vi "DAQ_AI_Chans.vi"(3 "error in":errorcluster, 5 "DAQ Settings":T1={"Shutters Settings"=[{"Name"="Shutter 1", "DAQ Channel/line"="Dev1/port0/line0", "Active"=FALSE}, {"Name"="Shutter 2", "DAQ Channel/line"="Dev1/port0/line1", "Active"=FALSE}], "Shutter Task"="", "Acquire Settings"=[], "AI Task"="", "Sample mode"=10178, "Number of Samples"=0, "Rate"=0.0, "AI Name"="", "DO Name"=""} {"Sample mode" items=["Finite Samples"=10178, "Continuous Samples"=10123, "Hardware Timed Single Point"=12522]; "Acquire Settings"."input terminal configuration" items=["default"=-1, "RSE"=10083, "NRSE"=10078, "Differential"=10106, "Pseudodifferential"=12529]}) -> (0 "error out":errorcluster, 2 "Acquire Out":refnum<k21>)   [LabVIEW 2020]
uses:
  Type defs/DAQ_set_Ctrl.ctl
  Type defs/DAQ_Shutter_Ctrl.ctl
  Type defs/DAQ_AI_Ctrl.ctl
  <vilib>/DAQmx/create/channels.llb/DAQmx Create Channel (AI-Voltage-Basic).vi
  <vilib>/DAQmx/configure/timing.llb/DAQmx Timing (Sample Clock).vi
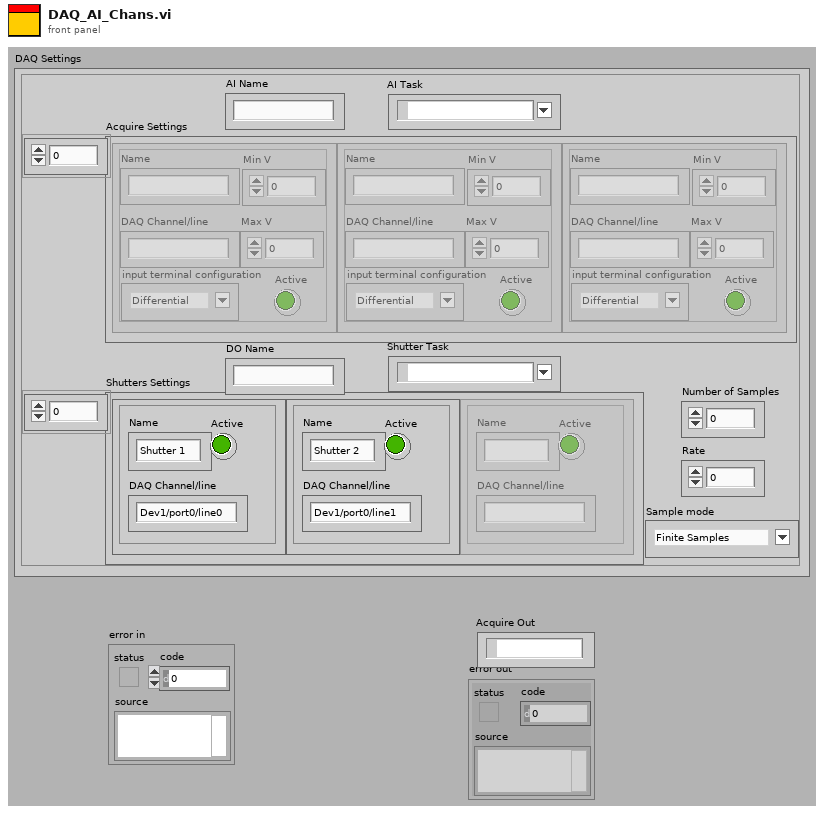
[diagram p1: front panel]
types:
  T1 = typedef "DAQ_set_Ctrl.ctl" = cluster{"Shutters Settings":T2[], "Shutter Task":refnum<k21>, "Acquire Settings":T3[], "AI Task":refnum<k21>, "Sample mode":i32, "Number of Samples":i32, "Rate":dbl, "AI Name":string, "DO Name":string}
  T2 = typedef "DAQ_Shutter_Ctrl.ctl" = cluster{"Name":string, "DAQ Channel/line":string, "Active":bool}
  T3 = typedef "DAQ_AI_Ctrl.ctl" = cluster{"Name":string, "DAQ Channel/line":string, "Max V":dbl, "Min V":dbl, "input terminal configuration":i32, "Active":bool}
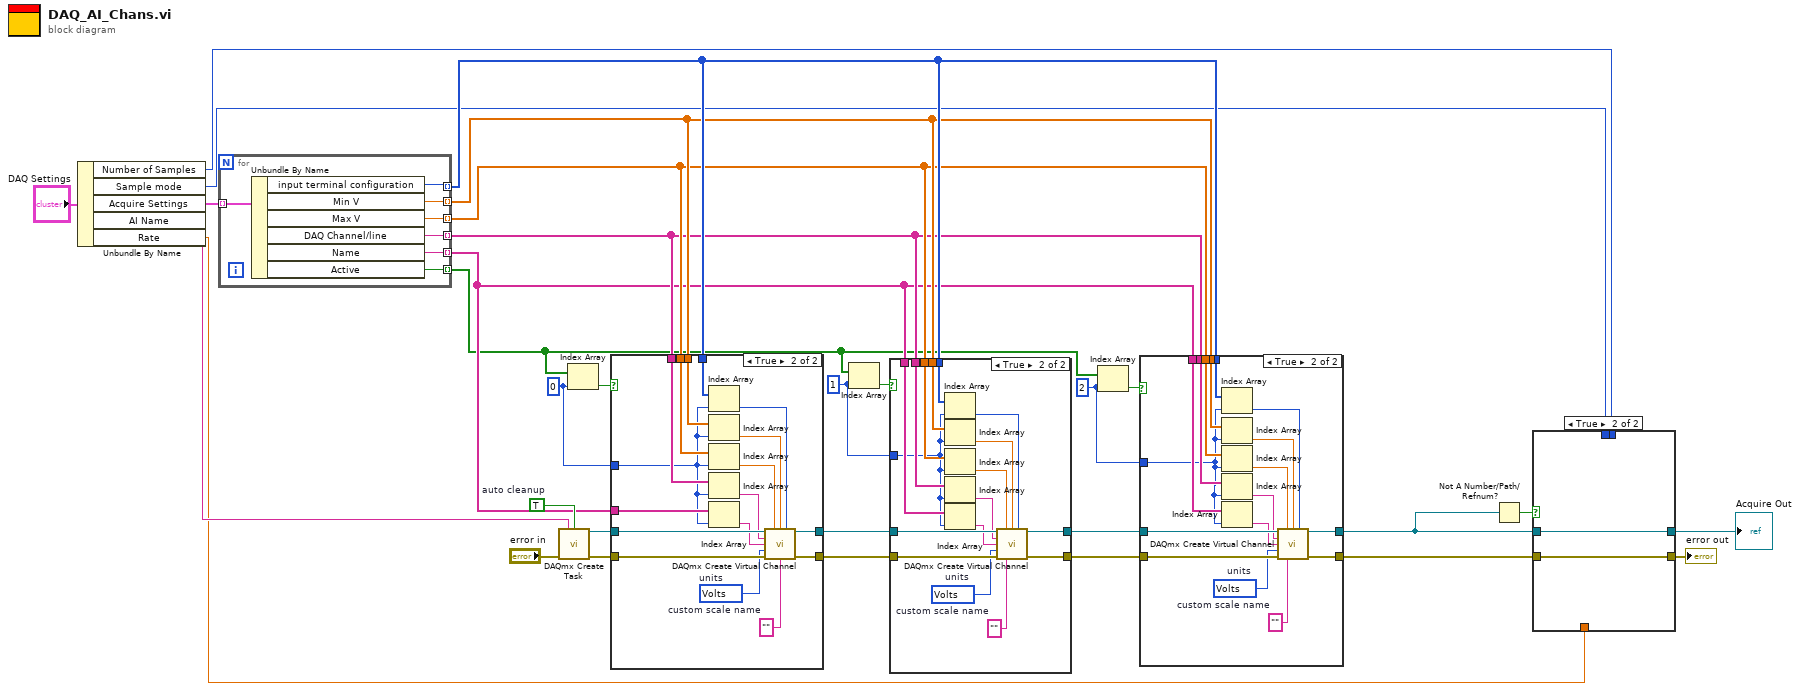
[diagram p0: block diagram]
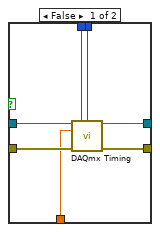
[diagram p2: hidden frame]
diagram:
  w15 = 2 ("index")
  w17 = 1 ("index")
  w19 = 0 ("index")
  w29 = TRUE  # auto cleanup
  n1 = Unbundle By Name("DAQ Settings") -> ("Number of Samples"=w4:i32, "Sample mode"=w3:i32, "Acquire Settings"=w13:T3[], "AI Name"=w6:string, "Rate"=w5:dbl)
  n2 = for {
    tunnel: w13 -> [w38] mode=indexing
    tunnel: [w37] -> w12 mode=indexing
    tunnel: [w36] -> w11 mode=indexing
    tunnel: [w35] -> w10 mode=indexing
    tunnel: [w34] -> w9 mode=indexing
    tunnel: [w33] -> w8 mode=indexing
    tunnel: [w32] -> w7 mode=indexing
    n3 = Unbundle By Name(w38) -> ("input terminal configuration"=w37:i32, "Min V"=w36:dbl, "Max V"=w35:dbl, "DAQ Channel/line"=w34:string, "Name"=w33:string, "Active"=w32:bool)
  }
  n4 = call <vilib>:"DAQmx Create Task.vi"("new task name"=w6, "auto cleanup"=w29, "error in"="error in") -> ("task out"=w28:refnum<k21>, "error out"=w30:errorcluster)  [unwired: 11 in]
  n5 = Index Array(array=w7, index=w19) -> (element=w20:bool)
  n6 = case shown="True" w20 {
    tunnel: w30 -> [w39 w57]
    tunnel: w28 -> [w40 w56]
    tunnel: [w39 w54] -> w27
    tunnel: [w40 w52] -> w26
    tunnel: w9 -> [_ w49]
    tunnel: w8 -> [_ w48]
    tunnel: w12 -> [_ w47]
    tunnel: w11 -> [_ w45]
    tunnel: w10 -> [_ w43]
    tunnel: w19 -> [_ w41]
    frame False {
    }
    frame True {
      w53 = 10348 items=["Volts"=10348, "From Custom Scale"=10065]  # units
      w55 = ""  # custom scale name
      n7 = Index Array(array=w47, index=w41) -> (element=w46:i32)
      n8 = Index Array(array=w45, index=w41) -> (element=w44:dbl)
      n9 = Index Array(array=w43, index=w41) -> (element=w42:dbl)
      n10 = Index Array(array=w49, index=w41) -> (element=w50:string)
      n11 = Index Array(array=w48, index=w41) -> (element=w51:string)
      n12 = call-poly <vilib>:"DAQmx Create Virtual Channel.vi"("task in"=w56, "maximum value"=w42, "minimum value"=w44, "input terminal configuration"=w46, "physical channels"=w50, "name to assign"=w51, "units"=w53, "error in"=w57, "custom scale name"=w55) -> ("task out"=w52:refnum<k21>, "error out"=w54:errorcluster)  [unwired: 5 in]
    }
  }
  n13 = Index Array(array=w7, index=w17) -> (element=w18:bool)
  n14 = case shown="True" w18 {
    tunnel: w27 -> [w59 w76]
    tunnel: w26 -> [w58 w75]
    tunnel: [w59 w73] -> w25
    tunnel: [w58 w71] -> w24
    tunnel: w9 -> [_ w68]
    tunnel: w8 -> [_ w67]
    tunnel: w12 -> [_ w66]
    tunnel: w11 -> [_ w64]
    tunnel: w10 -> [_ w63]
    tunnel: w17 -> [_ w60]
    frame False {
    }
    frame True {
      w72 = 10348 items=["Volts"=10348, "From Custom Scale"=10065]  # units
      w74 = ""  # custom scale name
      n15 = Index Array(array=w66, index=w60) -> (element=w65:i32)
      n16 = Index Array(array=w64, index=w60) -> (element=w62:dbl)
      n17 = Index Array(array=w63, index=w60) -> (element=w61:dbl)
      n18 = Index Array(array=w68, index=w60) -> (element=w69:string)
      n19 = Index Array(array=w67, index=w60) -> (element=w70:string)
      n20 = call-poly <vilib>:"DAQmx Create Virtual Channel.vi"("task in"=w75, "maximum value"=w61, "minimum value"=w62, "input terminal configuration"=w65, "physical channels"=w69, "name to assign"=w70, "units"=w72, "error in"=w76, "custom scale name"=w74) -> ("task out"=w71:refnum<k21>, "error out"=w73:errorcluster)  [unwired: 5 in]
    }
  }
  n21 = Index Array(array=w7, index=w15) -> (element=w16:bool)
  n22 = case shown="True" w16 {
    tunnel: w25 -> [w77 w95]
    tunnel: w24 -> [w78 w94]
    tunnel: [w77 w92] -> w23
    tunnel: [w78 w90] -> w2
    tunnel: w9 -> [_ w89]
    tunnel: w8 -> [_ w88]
    tunnel: w12 -> [_ w85]
    tunnel: w11 -> [_ w83]
    tunnel: w10 -> [_ w81]
    tunnel: w15 -> [_ w79]
    frame False {
    }
    frame True {
      w91 = 10348 items=["Volts"=10348, "From Custom Scale"=10065]  # units
      w93 = ""  # custom scale name
      n23 = Index Array(array=w85, index=w79) -> (element=w84:i32)
      n24 = Index Array(array=w83, index=w79) -> (element=w82:dbl)
      n25 = Index Array(array=w81, index=w79) -> (element=w80:dbl)
      n26 = Index Array(array=w89, index=w79) -> (element=w87:string)
      n27 = Index Array(array=w88, index=w79) -> (element=w86:string)
      n28 = call-poly <vilib>:"DAQmx Create Virtual Channel.vi"("task in"=w94, "maximum value"=w80, "minimum value"=w82, "input terminal configuration"=w84, "physical channels"=w87, "name to assign"=w86, "units"=w91, "error in"=w95, "custom scale name"=w93) -> ("task out"=w90:refnum<k21>, "error out"=w92:errorcluster)  [unwired: 5 in]
    }
  }
  n29 = Not A Number/Path/Refnum?(number/path/refnum=w2) -> (NaN/Path/Refnum?=w1:bool)
  n30 = case shown="True" w1 {
    tunnel: w23 -> [w102 w103]
    tunnel: [w101 w103] -> w22
    tunnel: [w100 w104] -> w21
    tunnel: w5 -> [w99 _]
    tunnel: w4 -> [w98 _]
    tunnel: w3 -> [w97 _]
    tunnel: w2 -> [w96 w104]
    frame False {
      n31 = call-poly <vilib>:"DAQmx Timing.vi"("task/channels in"=w96, "sample mode"=w97, "samples per channel"=w98, "rate"=w99, "error in"=w102) -> ("task out"=w100:refnum<k21>, "error out"=w101:errorcluster)  [unwired: 9 in]
    }
    frame True {
    }
  }
  "error out" <- w22
  "Acquire Out" <- w21
